vi "Write_CubeLiftCommand.vi"(8 "error in (no error)":errorcluster, 10 "Cube Lift Command":T1, 11 "CubeLiftData in":refnum<class "CubeLiftData.lvclass">) -> (0 "error out":errorcluster, 3 "CubeLiftData out":refnum<class "CubeLiftData.lvclass">)   [LabVIEW 2017, in "CubeLiftData.lvclass"]
uses:
  CubeLiftData.lvclass
  Team-code/CubeLiftCommand.ctl
  CubeLiftData.lvclass/CubeLiftData.ctl
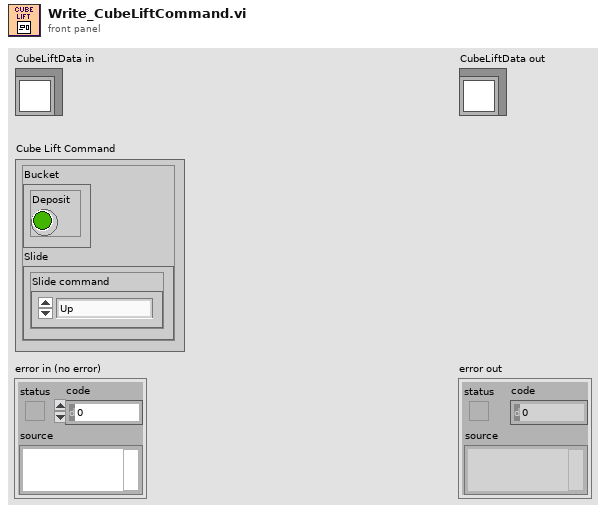
[diagram p1: front panel]
types:
  T1 = typedef "CubeLiftData.lvclass/CubeLiftCommand.ctl" = cluster{"Bucket":cluster{"Deposit":bool}, "Slide":cluster{"Slide command":enum16{"Up", "Down", "Stationary"}}}
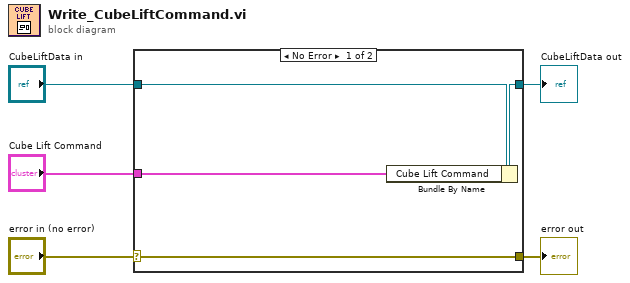
[diagram p0: block diagram]
diagram:
  n1 = case shown="No Error" "error in (no error)" {
    selector: "error in (no error)" -> [w9 w10]
    tunnel: [w9 w10] -> w4
    tunnel: [w7 w11] -> w2
    tunnel: "CubeLiftData in" -> [w8 w11]
    tunnel: "Cube Lift Command" -> [w6 _]
    frame No Error {
      n2 = Bundle By Name(cluster=w8, "Cube Lift Command"=w6) -> (w7:refnum<class "CubeLiftData.lvclass">)
    }
    frame Error {
    }
  }
  "error out" <- w4
  "CubeLiftData out" <- w2
